vi "Update Wave.vi"(8 "error in (no error)":errorcluster, 10 "wave":waveform(dbl)[](array[waveform]), 11 "[V] Waveform in":refnum<class "[V] Waveform.lvclass">) -> (0 "error out":errorcluster, 3 "[V] Waveform out":refnum<class "[V] Waveform.lvclass">)   [LabVIEW 2020, in "[V] Waveform.lvlib" / "[V] Waveform.lvclass"]
uses:
  [V] Waveform.lvclass
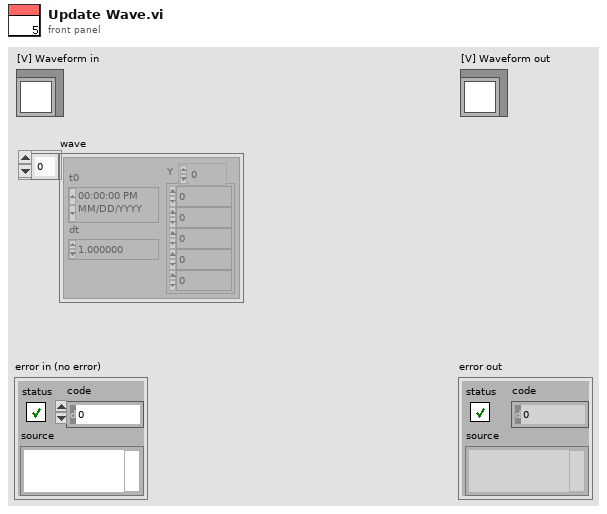
[diagram p1: front panel]
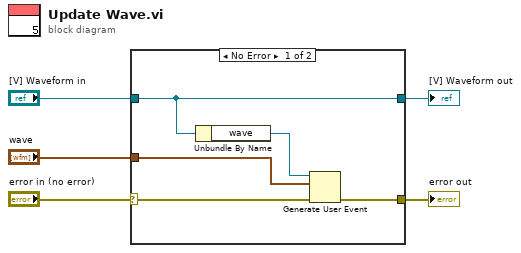
[diagram p0: block diagram]
diagram:
  n1 = case shown="No Error" "error in (no error)" {
    selector: "error in (no error)" -> [w9 w12]
    tunnel: [w6 w12] -> w4
    tunnel: [w10 w11] -> w2
    tunnel: "[V] Waveform in" -> [w10 w11]
    tunnel: "wave" -> [w7 _]
    frame No Error {
      n2 = Unbundle By Name(w10) -> ("wave"=w8:refnum<user-event>)
      n3 = Generate User Event(user event=w8, event data cluster=w7, error in=w9) -> (error out=w6:errorcluster)  [unwired: 1 in, 1 out]
    }
    frame Error {
    }
  }
  "error out" <- w4
  "[V] Waveform out" <- w2
